vi "Global cuenta erroes.vi"() -> ()   [LabVIEW 2019]
uses:
  global erroes cluster.ctl
panel:
  out "Errores":T1
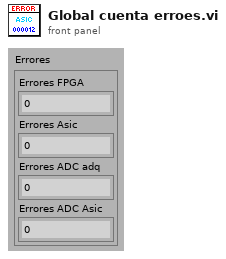
[diagram p1: front panel]
types:
  T1 = typedef "global erroes cluster.ctl" = cluster{"Errores FPGA":i32, "Errores Asic":i32, "Errores ADC adq":i32, "Errores ADC Asic":i32}
diagram:
